vi "Generate Key.vi"   [LabVIEW 2021]
uses:
  AES/AES.lvclass
  RSA/RSA.lvclass
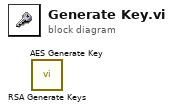
[diagram p0: block diagram]
diagram:
  n1 = call "RSA Generate Keys.vi"() -> ()  [unwired: 8 in, 4 out]
  n2 = call "AES Generate Key.vi"() -> ()  [unwired: 8 in, 4 out]
